vi "Emballage_mail_expedition_V141010.vi"(1 "Tableau Config email":string[][](array[string]), 2 "Article":string) -> (0 "Tab_Email_expedition":string[](array[string]))   [LabVIEW 2020]
panel:
  # "Produit complet ou division"
  # "email fin d'emballage"
  # "present"
  # "email de remplacement si absent"
  # "Email client en copie"
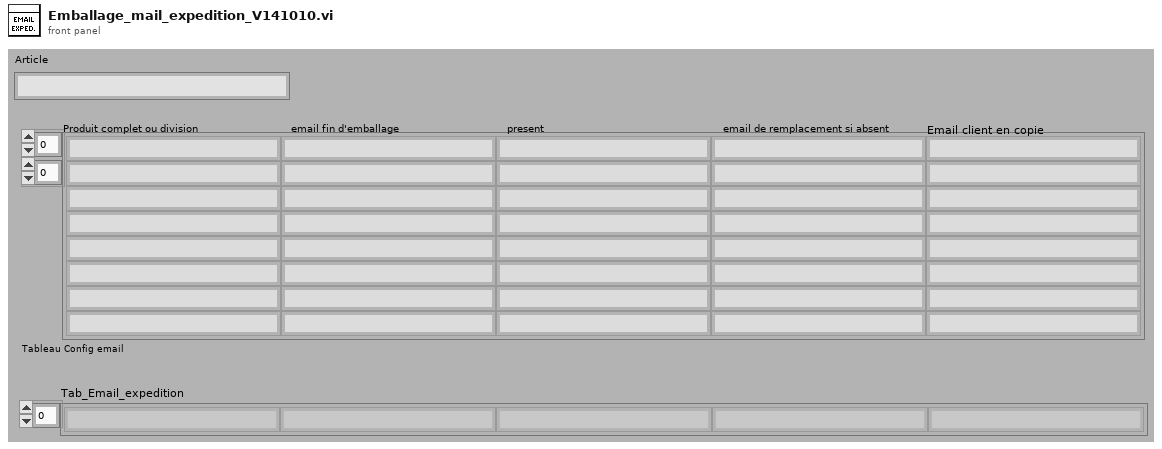
[diagram p1: front panel]
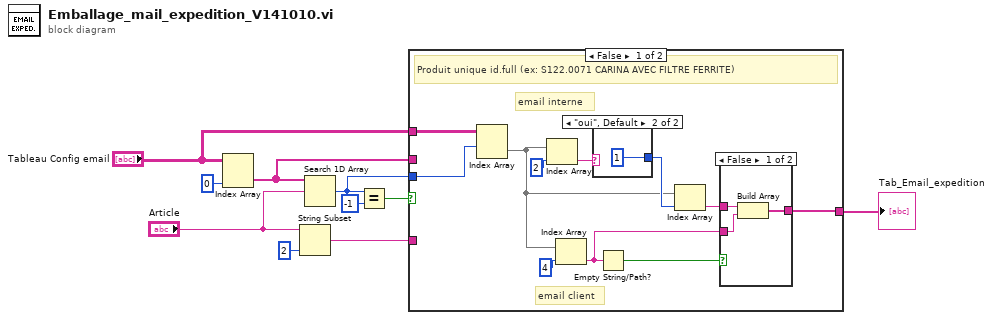
[diagram p0: block diagram]
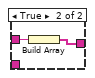
[diagram p2: hidden frame]
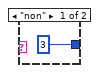
[diagram p3: hidden frame]
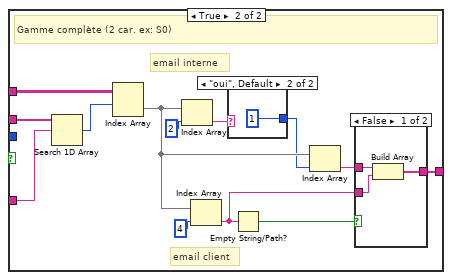
[diagram p4: hidden frame]
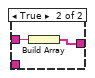
[diagram p5: hidden frame]
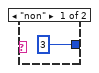
[diagram p6: hidden frame]
diagram:
  n1 = Index Array(array="Tableau Config email", index (col)=0 ("indice désactivé (col)")) -> (element=w4:string[])  [unwired: 1 in]
  n2 = String Subset(string="Article", length (rest)=2 ("longueur (reste)")) -> (substring=w5:string)  [unwired: 1 in]
  n3 = Search 1D Array(1D array=w4, element="Article") -> (index of element=w3:i32)  [unwired: 1 in]
  n4 = Equal?(x=w3, y=-1) -> (x = y?=w8:bool)
  n5 = case shown="False" w8 {
    tunnel: w5 -> [_ w41]
    tunnel: w4 -> [_ w40]
    tunnel: "Tableau Config email" -> [w21 w39]
    tunnel: w3 -> [w20 _]
    tunnel: [w11 w29] -> w1
    frame False {
      # "email interne"
      # "email client"
      # "Produit unique id.full (ex: S122.0071 CARINA AVEC FILTRE FERRITE)"
      n6 = Index Array(array=w21, index (row)=w20) -> (element=w12:string[])  [unwired: 1 in]
      n7 = Index Array(array=w12, index=2 ("indice")) -> (element=w18:string)
      n8 = Index Array(array=w12, index=4 ("indice")) -> (element=w13:string)
      n9 = case shown="\"oui\", Default" w18 {
        tunnel: [3 ("indice") 1 ("indice")] -> w16
        frame "non" {
        }
        frame "oui", Default {
        }
      }
      n10 = Empty String/Path?(string/path=w13) -> (empty?=w14:bool)
      n11 = Index Array(array=w12, index=w16) -> (element=w15:string)
      n12 = case shown="False" w14 {
        tunnel: w15 -> [w24 w26]
        tunnel: w13 -> [w23 _]
        tunnel: [w22 w25] -> w11
        frame False {
          n13 = Build Array(w24, w23) -> (w22:string[])
        }
        frame True {
          n14 = Build Array(w26) -> (w25:string[])
        }
      }
    }
    frame True {
      # "email interne"
      # "email client"
      # "Gamme complète (2 car. ex: S0)"
      n15 = Search 1D Array(1D array=w40, element=w41) -> (index of element=w38:i32)  [unwired: 1 in]
      n16 = Index Array(array=w39, index (row)=w38) -> (element=w34:string[])  [unwired: 1 in]
      n17 = Index Array(array=w34, index=2 ("indice")) -> (element=w36:string)
      n18 = Index Array(array=w34, index=4 ("indice")) -> (element=w30:string)
      n19 = case shown="\"oui\", Default" w36 {
        tunnel: [3 ("indice") 1 ("indice")] -> w33
        frame "non" {
        }
        frame "oui", Default {
        }
      }
      n20 = Empty String/Path?(string/path=w30) -> (empty?=w31:bool)
      n21 = Index Array(array=w34, index=w33) -> (element=w32:string)
      n22 = case shown="False" w31 {
        tunnel: w32 -> [w44 w46]
        tunnel: w30 -> [w43 _]
        tunnel: [w42 w45] -> w29
        frame False {
          n23 = Build Array(w44, w43) -> (w42:string[])
        }
        frame True {
          n24 = Build Array(w46) -> (w45:string[])
        }
      }
    }
  }
  "Tab_Email_expedition" <- w1
